vi "CAN Set Schedule.vi"(5 "MsgTabNum":u8, 6 "pSendTimes":u16, 7 "pMsgNum":string, 9 "pCanMsgTab":T1, 10 "CANIndex":u8, 11 "DevHandle":i32) -> (1 "pCanMsgTab out":T1, 2 "function return":i32, 3 "pMsgNum out":string, 4 "pSendTimes out":u16)   [LabVIEW 2010, in "usb2can.lvlib"]
doc: "int WINAPI CAN_SetSchedule(int DevHandle, unsigned char CANIndex, CAN_MSG *pCanMsgTab,unsigned char *pMsgNum,unsigned short *pSendTimes,unsigned char MsgTabNum);"
uses:
  usb2can.lvlib
  USB2XXX/trunk/USB2XXX/USB2XXX/vs2019/Release/USB2XXX.dll
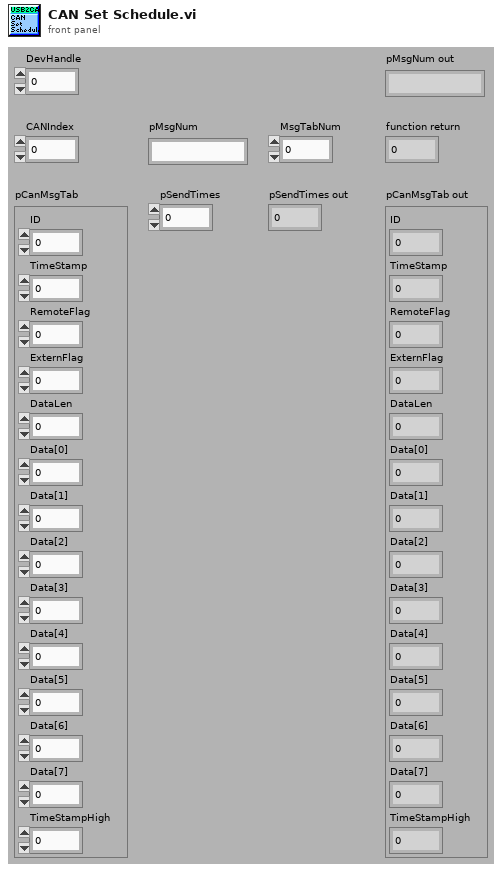
[diagram p1: front panel]
types:
  T1 = cluster{"ID":u32, "TimeStamp":u32, "RemoteFlag":u8, "ExternFlag":u8, "DataLen":u8, "Data[0]":u8, "Data[1]":u8, "Data[2]":u8, "Data[3]":u8, "Data[4]":u8, "Data[5]":u8, "Data[6]":u8, "Data[7]":u8, "TimeStampHigh":u8}
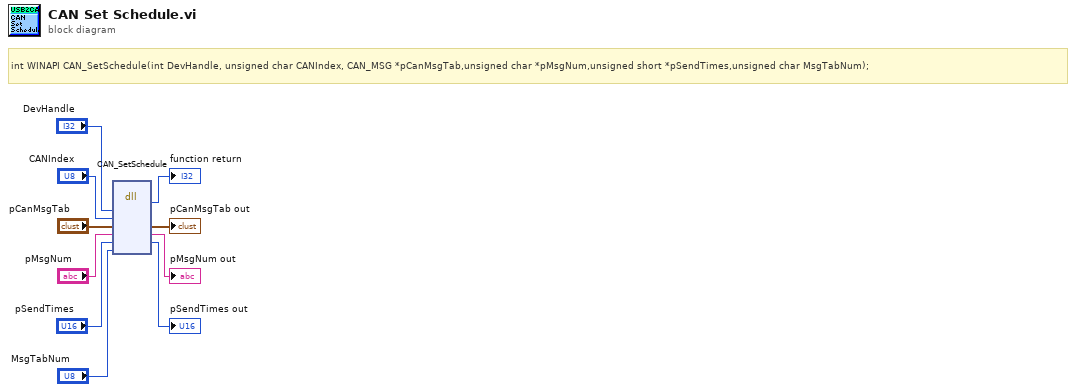
[diagram p0: block diagram]
diagram:
  # "int WINAPI CAN_SetSchedule(int DevHandle, unsigned char CANIndex, CAN_MSG *pCanMsgTab,unsigned char *pMsgNum,unsigned short *pSendTimes,unsigned char MsgTabNum);"
  n1 = dll-call lib="E:/Projects/USB2XXX/trunk/USB2XXX/USB2XXX/vs2019/Release/USB2XXX.*" fn="CAN_SetSchedule"("DevHandle"="DevHandle", "CANIndex"="CANIndex", "pCanMsgTab"="pCanMsgTab", "pMsgNum"="pMsgNum", "pSendTimes"="pSendTimes", "MsgTabNum"="MsgTabNum") -> (→"function return":i32, "pCanMsgTab"=→"pCanMsgTab out":T1, "pMsgNum"=→"pMsgNum out":string, "pSendTimes"=→"pSendTimes out":u16)  [unwired: 6 in, 2 out]
